vi "Stimulus.Open.vi"(8 "error in (no error)":errorcluster, 11 "State Variables":T1={"NIVS.BaseLogPath"=path "", "NIVS.SystemDefinitionFile"=path "", "NIVS.Events"={"SequenceEvent"=refnum, "SystemChangeEvent"=refnum, "WorkspaceEvent"=refnum}, "NIVS.SequenceState"=enum."Idle", "NIVS.GatewayIPAddress"="", "NIVS.DataLogSpecRef"=refnum, "NIVS.DataLogManagerRef"=refnum, "NIVS.LogSessionGUID"="", "NIVS.WorkspaceManager"=refnum, "NIVS.Deployed"=FALSE, "NIVS.ProfileRef"=refnum, "NIVS.ProfileCallback"=refnum, "NIVS.SystemStateRefs"={"CustDatRef"=refnum, "EvtRef"=refnum}, "UI.Abort"=refnum, "UI.Pause"=refnum, "UI.EnableLogging"=refnum, "UI.Start"=refnum, "UI.LogChannels"=refnum, "UI.StartIteration"=refnum, "UI.StartStep"=refnum, "UI.Sequence"=refnum, "UI.PreviewMode"=refnum, "UI.Graph"=refnum, "UI.BaseFileName"=refnum, "UI.Profiles"=refnum, "UI.CurrentStep"=refnum, "UI.CurrentIteration"=refnum, "UI.TotalIterations"=refnum, "Sequence.AbortChannel"="", "Sequence.StepInfoChannel"="", "Sequence.Iterations"=0, "Sequence.IterationInfoChannel"="", "Sequence.#ofColumns"=0, "Events.State"=refnum, "Events.Test Result"=refnum, "Events.Progress"=refnum, "INI.Settings"={"Build Location"=path "C:/Simple Sequence Editor/SequenceRepo", "LoggingLocation"=path ""}, "UI.Skip"=refnum, "Sequence.SkipChannel"="", "Restart.Path"=path ""}) -> (0 "error out":errorcluster, 3 "State Variables":T1={"NIVS.BaseLogPath"=path "", "NIVS.SystemDefinitionFile"=path "", "NIVS.Events"={"SequenceEvent"=refnum, "SystemChangeEvent"=refnum, "WorkspaceEvent"=refnum}, "NIVS.SequenceState"=enum."Idle", "NIVS.GatewayIPAddress"="", "NIVS.DataLogSpecRef"=refnum, "NIVS.DataLogManagerRef"=refnum, "NIVS.LogSessionGUID"="", "NIVS.WorkspaceManager"=refnum, "NIVS.Deployed"=FALSE, "NIVS.ProfileRef"=refnum, "NIVS.ProfileCallback"=refnum, "NIVS.SystemStateRefs"={"CustDatRef"=refnum, "EvtRef"=refnum}, "UI.Abort"=refnum, "UI.Pause"=refnum, "UI.EnableLogging"=refnum, "UI.Start"=refnum, "UI.LogChannels"=refnum, "UI.StartIteration"=refnum, "UI.StartStep"=refnum, "UI.Sequence"=refnum, "UI.PreviewMode"=refnum, "UI.Graph"=refnum, "UI.BaseFileName"=refnum, "UI.Profiles"=refnum, "UI.CurrentStep"=refnum, "UI.CurrentIteration"=refnum, "UI.TotalIterations"=refnum, "Sequence.AbortChannel"="", "Sequence.StepInfoChannel"="", "Sequence.Iterations"=0, "Sequence.IterationInfoChannel"="", "Sequence.#ofColumns"=0, "Events.State"=refnum, "Events.Test Result"=refnum, "Events.Progress"=refnum, "INI.Settings"={"Build Location"=path "C:/Simple Sequence Editor/SequenceRepo", "LoggingLocation"=path ""}, "UI.Skip"=refnum, "Sequence.SkipChannel"="", "Restart.Path"=path ""})   [LabVIEW 2013, in "Simple Sequence Tools - Execution.lvlib"]
uses:
  Simple Sequence Tools - Execution.lvlib
  Types/Main.StateVariables.ctl
  Types/Execute.UserEventRefs.ctl
  <vilib>/NI Veristand/Execution/Workspace/SystemStateRegEventRef.ctl
  Types/Execution.SequenceState.ctl
  <vilib>/NI Veristand/Execution/DataLogging/DataLoggingSpecification Ref.ctl
  NationalInstruments.VeriStand.ClientAPI
  <vilib>/NI Veristand/Execution/DataLogging/IDataLogging Ref.ctl
  <vilib>/NI Veristand/Execution/Workspace/WorkspaceAPI.ctl
  NationalInstruments.VeriStand.RealTimeSequenceDefinitionApi
  <vilib>/NI Veristand/Execution/Workspace/SystemStateEventRef.ctl
  Shared/Types/INI.Settings
  NationalInstruments.VeriStand.DataTypes
  <vilib>/NI Veristand/Execution/DataLogging/File Conflict Operation.ctl
  Shared/SubVIs/Main.Constants.vi
  <vilib>/NI Veristand/Execution/DataLogging/New Data Logging Specification (TDMS).vi
  <vilib>/NI Veristand/Execution/DataLogging/Set Data Logging Rate (Target Rate).vi
  <vilib>/NI Veristand/Execution/DataLogging/Set Start Trigger (Start Immediately).vi
  Shared/Simple Sequence Tools - Shared.lvlib
  <vilib>/NI Veristand/Execution/DataLogging/NI_VS Data Logging API.lvlib
  <vilib>/NI Veristand/Execution/Workspace/NI_VS Workspace ExecutionAPI.lvlib
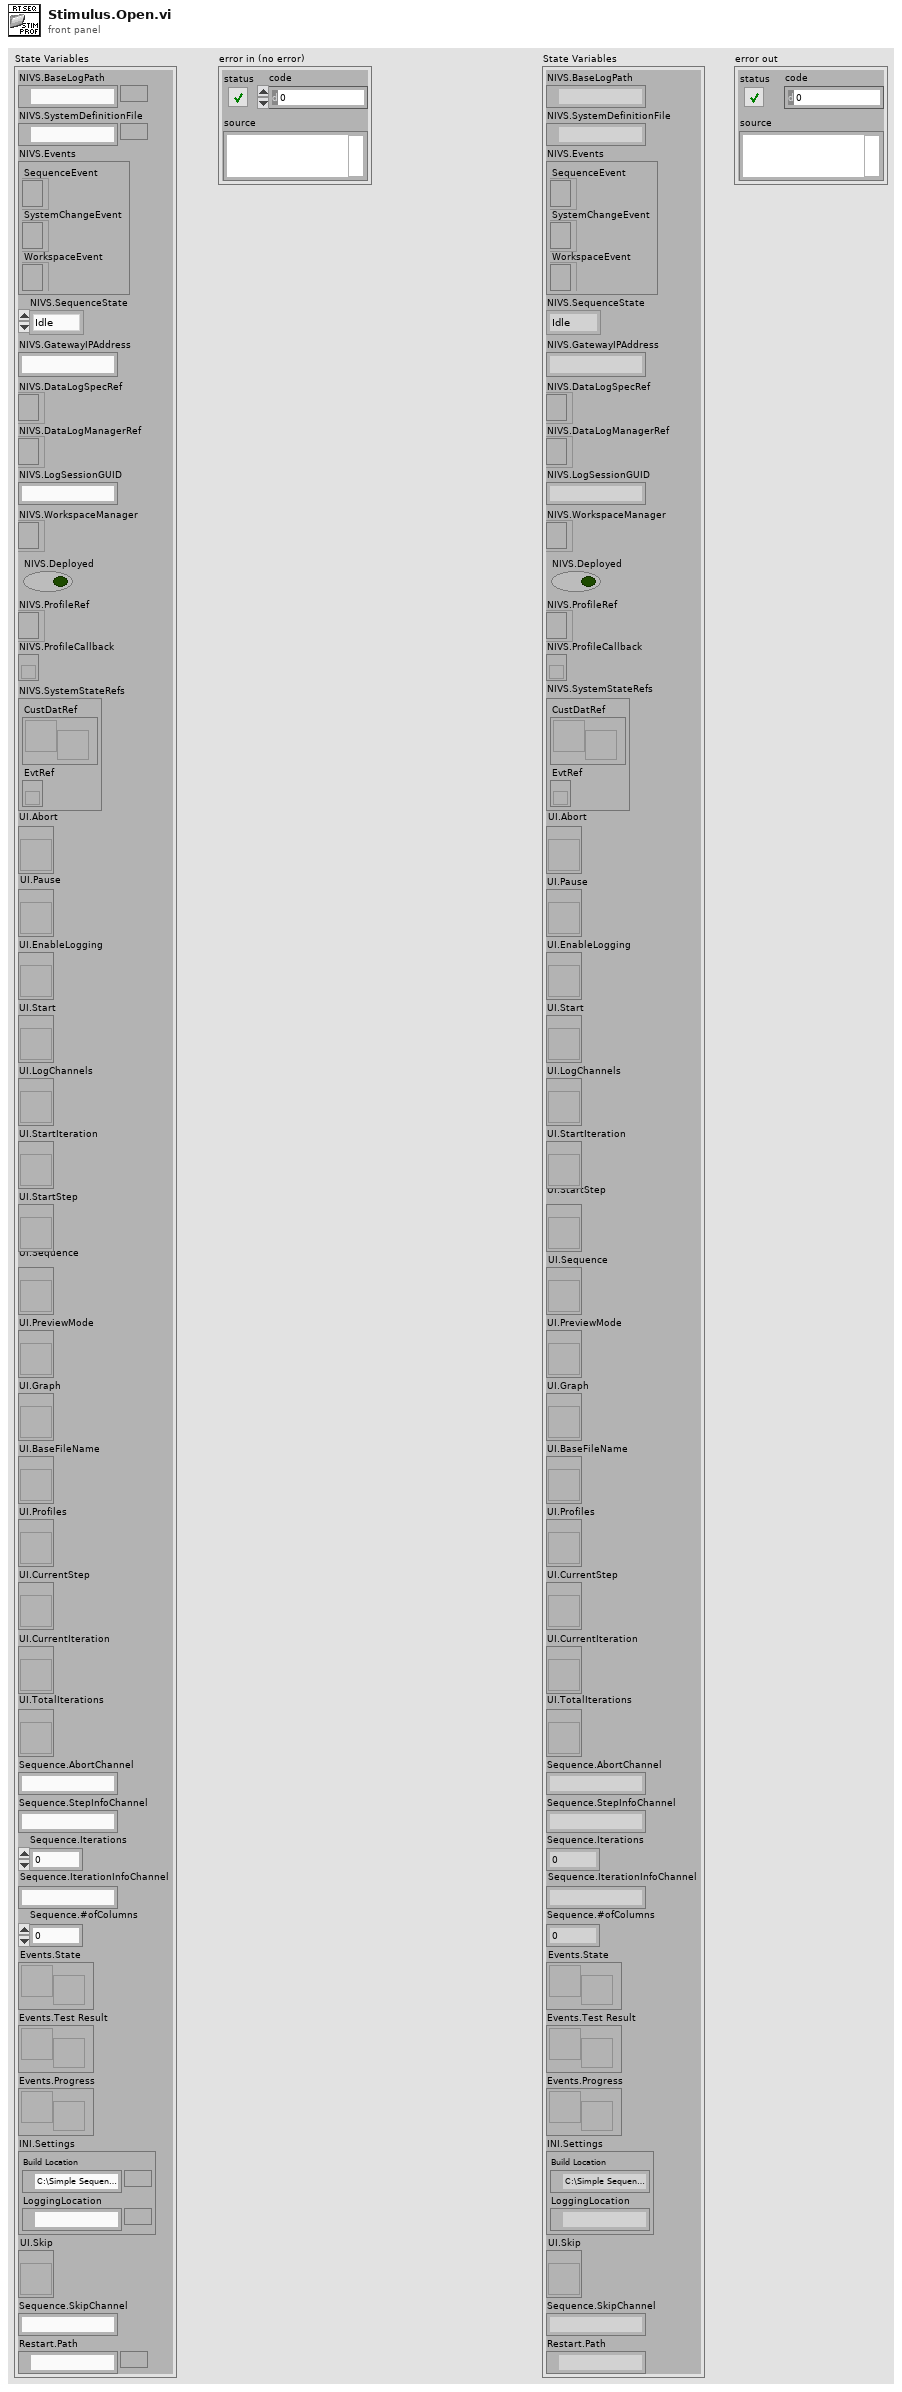
[diagram p1: front panel]
types:
  T1 = typedef "Simple Sequence Tools - Execution.lvlib/Main.StateVariables.ctl" = cluster{"NIVS.BaseLogPath":path, "NIVS.SystemDefinitionFile":path, "NIVS.Events":T2, "NIVS.SequenceState":T4, "NIVS.GatewayIPAddress":string, "NIVS.DataLogSpecRef":T5, "NIVS.DataLogManagerRef":T6, "NIVS.LogSessionGUID":string, "NIVS.WorkspaceManager":T7, "NIVS.Deployed":bool, "NIVS.ProfileRef":refnum<k24>, "NIVS.ProfileCallback":refnum<k27>, "NIVS.SystemStateRefs":T8, "UI.Abort":refnum<vi>, "UI.Pause":refnum<vi>, "UI.EnableLogging":refnum<vi>, "UI.Start":refnum<vi>, "UI.LogChannels":refnum<vi>, "UI.StartIteration":refnum<vi>, "UI.StartStep":refnum<vi>, "UI.Sequence":refnum<vi>, "UI.PreviewMode":refnum<vi>, "UI.Graph":refnum<vi>, "UI.BaseFileName":refnum<vi>, "UI.Profiles":refnum<vi>, "UI.CurrentStep":refnum<vi>, "UI.CurrentIteration":refnum<vi>, "UI.TotalIterations":refnum<vi>, "Sequence.AbortChannel":string, "Sequence.StepInfoChannel":string, "Sequence.Iterations":u32, "Sequence.IterationInfoChannel":string, "Sequence.#ofColumns":i32, "Events.State":refnum<user-event>, "Events.Test Result":refnum<user-event>, "Events.Progress":refnum<user-event>, "INI.Settings":T9, "UI.Skip":refnum<vi>, "Sequence.SkipChannel":string, "Restart.Path":path}
  T2 = typedef "Simple Sequence Tools - Execution.lvlib/Execute.UserEventRefs.ctl" = cluster{"SequenceEvent":refnum<event-registration>, "SystemChangeEvent":T3, "WorkspaceEvent":refnum<event-registration>}
  T3 = typedef "NI_VS Workspace ExecutionAPI.lvlib/SystemStateRegEventRef.ctl" = refnum<event-registration>
  T4 = typedef "Simple Sequence Tools - Execution.lvlib/Execution.SequenceState.ctl" = enum16{"Idle", "Initializing", "Running", "Paused", "Finalizing", "Complete"}
  T5 = typedef "NI_VS Data Logging API.lvlib/DataLoggingSpecification Ref.ctl" = refnum<k24>
  T6 = typedef "NI_VS Data Logging API.lvlib/IDataLogging Ref.ctl" = refnum<k24>
  T7 = typedef "NI_VS Workspace ExecutionAPI.lvlib/WorkspaceAPI.ctl" = refnum<k24>
  T8 = typedef "NI_VS Workspace ExecutionAPI.lvlib/SystemStateEventRef.ctl" = cluster{"CustDatRef":refnum<user-event>, "EvtRef":refnum<k27>}
  T9 = typedef "Simple Sequence Tools - Shared.lvlib/INI.Settings" = cluster{"Build Location":path, "LoggingLocation":path}
  T10 = typedef "Simple Sequence Tools - Execution.lvlib/Restart.Settings" = cluster{"LogFile":path, "Log Settings":T11[], "StimulusProfile":path, "StopIteration":u32, "StopStep":u32, "Log Channels":T15, "Base File Name":string, "Enable Logging":bool, "Profile":string}
  T11 = typedef "NI_VS Data Logging API.lvlib/TDMS Channel Group.ctl" = cluster{"Group Name":string, "Group Description":string, "Group Properties":T12[], "Channels":T13[], "Time Channel Options":T14, "Time Channel Name":string}
  T12 = typedef "NI_VS Data Logging API.lvlib/TDMS Property.ctl" = cluster{"Name":string, "Value":variant}
  T13 = typedef "NI_VS Data Logging API.lvlib/TDMS Channel.ctl" = cluster{"Channel Name":string, "Channel Path":string, "Channel Description":string, "Channel Properties":T12[]}
  T14 = typedef "NI_VS Data Logging API.lvlib/Time Channel Options.ctl" = enum16{"No Time Channel", "Absolute Time", "System Time", "System Time - Microseconds", "Absolute Time as Double"}
  T15 = typedef "Simple Sequence Tools - Execution.lvlib/Log.SelectedChannels.ctl" = enum16{"Channels (No System Channel)", "Aliases", "All"}
  T16 = typedef "NI_VS Data Logging API.lvlib/File Conflict Operation.ctl" = enum16{"Create Unique", "Append to Existing", "Overwrite"}
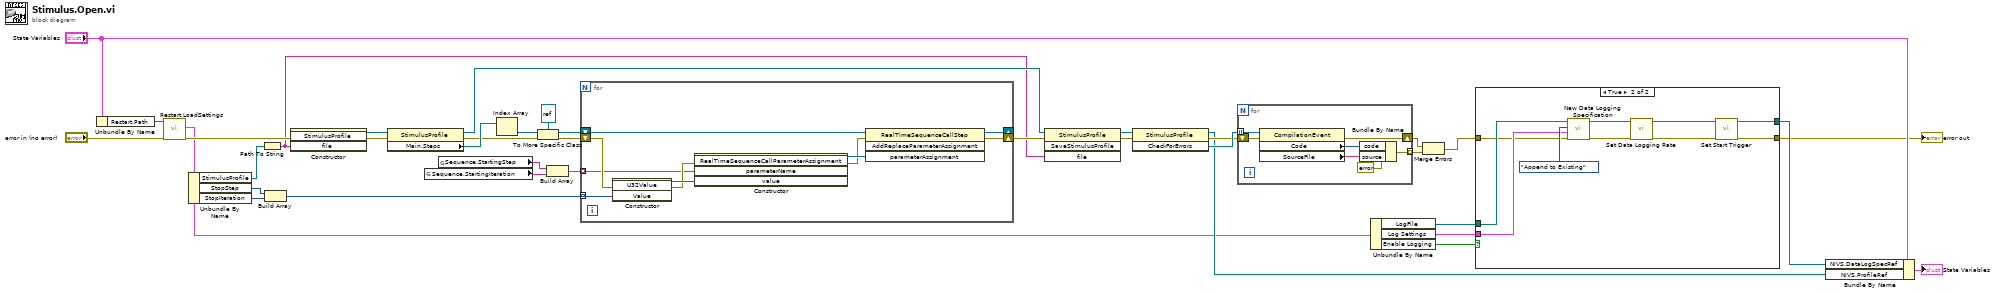
[diagram p0: block diagram]
diagram:
  n1 = Unbundle By Name("State Variables") -> ("Restart.Path"=w20:path)
  n2 = call "Restart.LoadSettings.vi"("error in"="error in (no error)", "datalog path (use dialog)"=w20) -> ("error out"=w9:errorcluster, "Restart Settings"=w5:T10)  [unwired: 7 in, 1 out]
  n3 = Unbundle By Name(w5) -> ("StimulusProfile"=w17:path, "StopStep"=w18:u32, "StopIteration"=w19:u32)
  n4 = Path To String(path=w17) -> (string=w6:string)
  n5 = Build Array(w18, w19) -> (w10:u32[])
  n6 = constructor class="StimulusProfile"(error in=w9, "file"=w6) -> (reference out=w35:refnum<k24>, error out=w34:errorcluster)  [unwired: 2 in, 2 out]
  n7 = property class="StimulusProfile"(reference=w35, error in=w34) -> (reference out=w25:refnum<k24>, error out=w13:errorcluster, "Main.Steps"=w16:refnum<k24>[])
  n8 = global read "Main.Constants.vi" "Sequence.StartingIteration"() -> (w26:string)
  n9 = global read "Main.Constants.vi" "Sequence.StartingStep"() -> (w27:string)
  n10 = Index Array(array=w16) -> (element=w15:refnum<k24>)  [unwired: 1 in]
  n11 = To More Specific Class(target class=refnum<k24> refnum ("new reference"), reference=w15, error in=w13) -> (specific class reference=w12:refnum<k24>, error out=w8:errorcluster)
  n12 = Build Array(w27, w26) -> (w11:string[])
  n13 = for {
    tunnel: w11 -> [w40] mode=indexing
    tunnel: w10 -> [w38] mode=indexing
    shift-right: [w45] -> _
    shift-left: w12 -> [w46]
    shift-right: [w47] -> w7
    shift-left: w8 -> [w41]
    n14 = constructor class="U32Value"(error in=w41, "Value"=w38) -> (reference out=w43:refnum<k24>, error out=w42:errorcluster)  [unwired: 2 in, 2 out]
    n15 = constructor class="RealTimeSequenceCallParameterAs"(error in=w42, "parameterName"=w40, "value"=w43) -> (reference out=w44:refnum<k24>, error out=w39:errorcluster)  [unwired: 2 in, 3 out]
    n16 = invoke class="RealTimeSequenceCallStep" method="AddReplaceParameterAssignment"(reference=w46, error in=w39, "parameterAssignment"=w44) -> (reference out=w45:refnum<k24>, error out=w47:errorcluster)  [unwired: 1 in, 2 out]
  }
  n17 = invoke class="StimulusProfile" method="SaveStimulusProfile"(reference=w25, error in=w7, "file"=w6) -> (reference out=w33:refnum<k24>, error out=w32:errorcluster)  [unwired: 1 in, 2 out]
  n18 = invoke class="StimulusProfile" method="CheckForErrors"(reference=w33, error in=w32) -> (reference out=w23:refnum<k24>, error out=w30:errorcluster, "CheckForErrors"=w31:refnum<k24>[])  [unwired: 1 in]
  n19 = for {
    tunnel: w31 -> [w54] mode=indexing
    tunnel: [w49] -> w28 mode=indexing
    shift-right: [w48] -> w29
    shift-left: w30 -> [w53]
    n20 = property class="CompilationEvent"(reference=w54, error in=w53) -> (error out=w48:errorcluster, "Code"=w51:i32, "SourceFile"=w50:string)  [unwired: 1 out]
    n21 = Bundle By Name(cluster=errorcluster {"status"=TRUE, "code"=0, "source"=""} ("error out"), "code"=w51, "source"=w50) -> (w49:errorcluster)
  }
  n22 = Unbundle By Name(w5) -> ("LogFile"=w3:path, "Log Settings"=w1:T11[], "Enable Logging"=w4:bool)
  n23 = Merge Errors(w29, w28) -> (w2:errorcluster)
  n24 = case shown="True" w4 {
    tunnel: w2 -> [w55 w56]
    tunnel: [w55 w60] -> w22
    tunnel: [_ w59] -> w24
    tunnel: w3 -> [_ w58]
    tunnel: w1 -> [_ w57]
    frame False {
    }
    frame True {
      n25 = call-poly <vilib>:"New Data Logging Specification.vi"("error in (no error)"=w56, "Channel Groups"=w57, "File Conflict Operation"=File_Conflict_Operation."Append to Existing", "Base Log File Path"=w58) -> ("error out"=w62:errorcluster, "Data Logging Specification Ref out"=w65:T5)  [unwired: 6 in]
      n26 = call-poly <vilib>:"Set Data Logging Rate.vi"("error in (no error)"=w62, "Data Logging Specification Ref in"=w65) -> ("error out"=w63:errorcluster, "Data Logging Specification Ref out"=w64:T5)  [unwired: 8 in]
      n27 = call-poly <vilib>:"Set Start Trigger.vi"("error in (no error)"=w63, "Data Logging Specification Ref in"=w64) -> ("error out"=w60:errorcluster, "Data Logging Specification Ref out"=w59:T5)  [unwired: 8 in]
    }
  }
  "error out" <- w22
  n28 = Bundle By Name(cluster="State Variables", "NIVS.DataLogSpecRef"=w24, "NIVS.ProfileRef"=w23) -> (→"State Variables":T1)
